vi "__Temp_Get.vi"(10 "Bias_LO_equip":T1={"Node address"=19, "CAN Interface"="CAN0", "Cartridge band"=10, "Slave Node in"={"Address"=0, "Serial Number"=[]}, "ObjHandle out"=0, "POL"=1, "sb"=1, "GPIB_SM (SIS S,V)"="24", "GPIB_DMM (SIS I)"="22", "GPIB_SM (MAG I) "="25", "GPIB_SG(LO)"="19", "GPIB_PW (PAMP) "="6", "GPIB_TMP1(8ch)"="12", "GPIB_TMP2(2ch)  "="13", "WCA_avg"=10, "Rsen"=10.0, "BiasModule"=0, "LOModule "=1, "WCA_LO_FREQ_SET"={"YTO Low freq. [GHz]"=14.42, "YTO High freq. [GHz]"=17.7, "Kvco"=1, "Lock Pol."=0, "SET LO FREQ"=72.5, "Multiplier"=6.0, "YTO (HEX)"=0, "YTO coarse( FREQ)"=25.0, "NULL PLL INTEGRATOR"=FALSE}, "Res for"=0} {"Res for" items=["none", "series res", "parallel res"]; "WCA_LO_FREQ_SET"."YTO coarse( FREQ)" min=25 max=150 step=0.0001 format="%.3f"; "WCA_LO_FREQ_SET"."Multiplier" min=3 max=6 step=3; "WCA_LO_FREQ_SET"."SET LO FREQ" min=25 max=150 step=0.0001 format="%.3f"; "WCA_LO_FREQ_SET"."Lock Pol." items=["Lower", "Upper"]; "WCA_LO_FREQ_SET"."Kvco" items=["7.5MHz/V", "15MHz/V"]; "WCA_LO_FREQ_SET"."YTO High freq. [GHz]" format="%.3f"; "WCA_LO_FREQ_SET"."YTO Low freq. [GHz]" format="%.3f"; "LOModule" items=["Manual", "B10Lab LO", "WCA LO"]; "BiasModule" items=["B10Lab Bias", "WCA BiasModule"]; "Slave Node in"."Serial Number" format="%.0x"; "Slave Node in"."Address" format="%.0x"; "Cartridge band" max=10 step=1; "Node address" format="%.0x"}) -> (0 "MixTemp":dbl=3.853, 2 "90/20K_temp":dbl=15.514, 3 "4K_Temp":dbl=3.005)   [LabVIEW 2017]
panel:
  out "error out":errorcluster caption="エラー出力"
  # "LO freq. [GHz]"
  # "YTO LOW\n/High Freq."
  # "ZERO Intgrtr"
  # "Node Address"
  # "Serial Number"
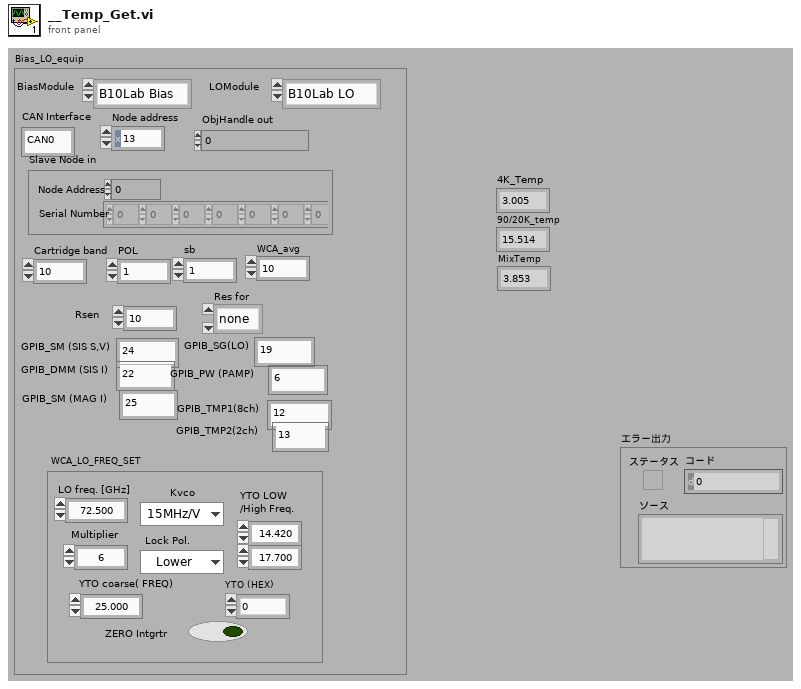
[diagram p1: front panel]
types:
  T1 = cluster{"Node address":u16, "CAN Interface":string, "Cartridge band":u32, "Slave Node in":cluster{"Address":i16, "Serial Number":i8[]}, "ObjHandle out":u32, "POL":u32, "sb":u32, "GPIB_SM (SIS S,V)":string, "GPIB_DMM (SIS I)":string, "GPIB_SM (MAG I) ":string, "GPIB_SG(LO)":string, "GPIB_PW (PAMP) ":string, "GPIB_TMP1(8ch)":string, "GPIB_TMP2(2ch)  ":string, "WCA_avg":i32, "Rsen":dbl, "BiasModule":u16, "LOModule ":u16, "WCA_LO_FREQ_SET":cluster{"YTO Low freq. [GHz]":sgl, "YTO High freq. [GHz]":sgl, "Kvco":u16, "Lock Pol.":u16, "SET LO FREQ":sgl, "Multiplier":sgl, "YTO (HEX)":u16, "YTO coarse( FREQ)":sgl, "NULL PLL INTEGRATOR":bool}, "Res for":u16}
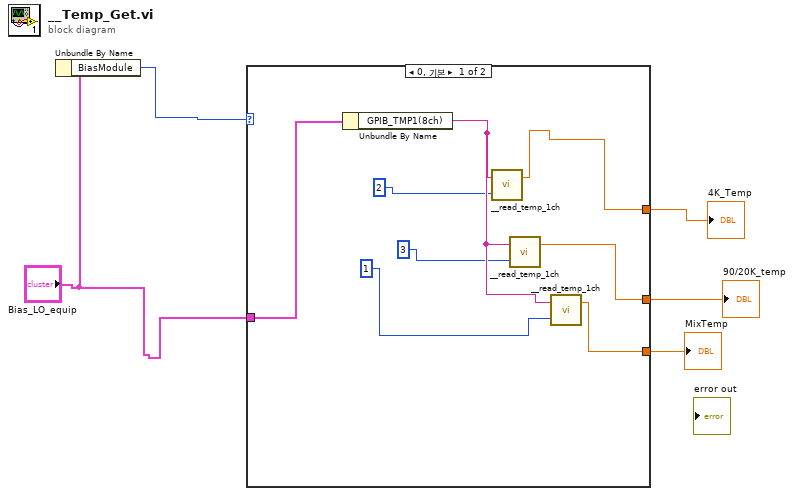
[diagram p0: block diagram]
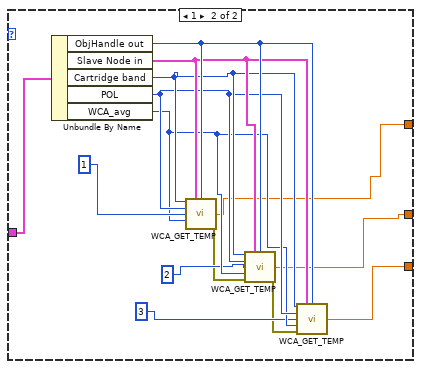
[diagram p2: hidden frame]
diagram:
  n1 = Unbundle By Name("Bias_LO_equip") -> ("BiasModule"=w3:u16)
  n2 = case shown="0, 기본" w3 {
    tunnel: "Bias_LO_equip" -> [w13 w27]
    tunnel: [w10 w14] -> w5
    tunnel: [w6 w15] -> w2
    tunnel: [w8 w18] -> w1
    frame 0, Default {
      n3 = Unbundle By Name(w13) -> ("GPIB_TMP1(8ch)"=w12:string)
      n4 = call "__read_temp_1ch.vi"("ch"=2, "GIPB番号"=w12) -> ("input A"=w10:dbl)  [unwired: 1 in]
      n5 = call "__read_temp_1ch.vi"("ch"=3, "GIPB番号"=w12) -> ("input A"=w6:dbl)  [unwired: 1 in]
      n6 = call "__read_temp_1ch.vi"("ch"=1, "GIPB番号"=w12) -> ("input A"=w8:dbl)  [unwired: 1 in]
    }
    frame 1 {
      n7 = Unbundle By Name(w27) -> ("ObjHandle out"=w25:u32, "Slave Node in"=w24:cluster{"Address":i16, "Serial Number":i8[]}, "Cartridge band"=w23:u32, "POL"=w22:u32, "WCA_avg"=w21:i32)
      n8 = call "WCA_GET_TEMP.vi"("Cartridge Band"=w23, "Slave Node in"=w24, "ObjHandle in"=w25, "POL"=w22, "No(1:4/p1,2:90/20,3:mix)"=1, "avg"=w21) -> ("get"=w14:dbl, "error out"=w16:errorcluster)  [unwired: 7 in, 1 out]
      n9 = call "WCA_GET_TEMP.vi"("Cartridge Band"=w23, "Slave Node in"=w24, "ObjHandle in"=w25, "POL"=w22, "No(1:4/p1,2:90/20,3:mix)"=2, "avg"=w21, "error in (no error)"=w16) -> ("get"=w15:dbl, "error out"=w17:errorcluster)  [unwired: 6 in, 1 out]
      n10 = call "WCA_GET_TEMP.vi"("Cartridge Band"=w23, "Slave Node in"=w24, "ObjHandle in"=w25, "POL"=w22, "No(1:4/p1,2:90/20,3:mix)"=3, "avg"=w21, "error in (no error)"=w17) -> ("get"=w18:dbl)  [unwired: 6 in, 2 out]
    }
  }
  "4K_Temp" <- w5
  "90/20K_temp" <- w2
  "MixTemp" <- w1
